vi "AddEntry.vi"(10 "Entry":string, 11 "Journal In":refnum<class "Journal.lvclass">) -> (2 "Count":i32, 3 "Journal Out":refnum<class "Journal.lvclass">)   [LabVIEW 2018, in "Journal.lvclass"]
uses:
  Journal.lvclass
  Journal.lvclass/Journal.ctl
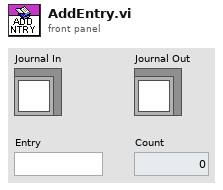
[diagram p1: front panel]
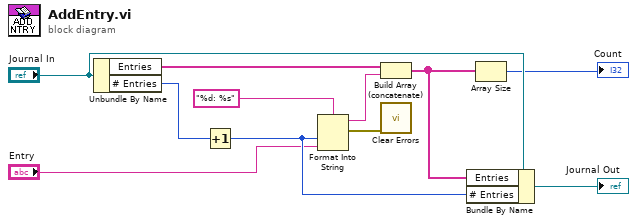
[diagram p0: block diagram]
diagram:
  n1 = Unbundle By Name("Journal In") -> ("Entries"=w9:string[], "# Entries"=w6:i32)
  n2 = Increment(x=w6) -> (x+1=w4:i32)
  n3 = Format Into String(format string="%d: %s", w4, "Entry") -> (resulting string=w2:string, error out=w1:errorcluster)  [unwired: 2 in]
  n4 = Build Array (concatenate)(w9, w2) -> (w8:string[])
  n5 = call <vilib>:"Clear Errors.vi"("error in (no error)"=w1) -> ()  [unwired: 5 in, 2 out]
  n6 = Bundle By Name(cluster="Journal In", "Entries"=w8, "# Entries"=w4) -> (→"Journal Out":refnum<class "Journal.lvclass">)
  n7 = Array Size(array=w8) -> (size(s)=→"Count":i32)
